vi "Remove INI Keys.vi"(8 "error in (no error)":errorcluster, 10 "Keys to remove":T1[](array[typedef]), 11 "INI file path":path) -> (0 "error out":errorcluster, 3 "Errors":string[](array[string]))   [LabVIEW 2016, in "RT Management.lvlib"]
doc: "Removes INI keys. If a key is the last one under a section and is removed, the section is left alone."
uses:
  RT Management.lvlib
  controls/INI key.ctl
  <vilib>/Utility/config.llb/NI_LVConfig.lvlib
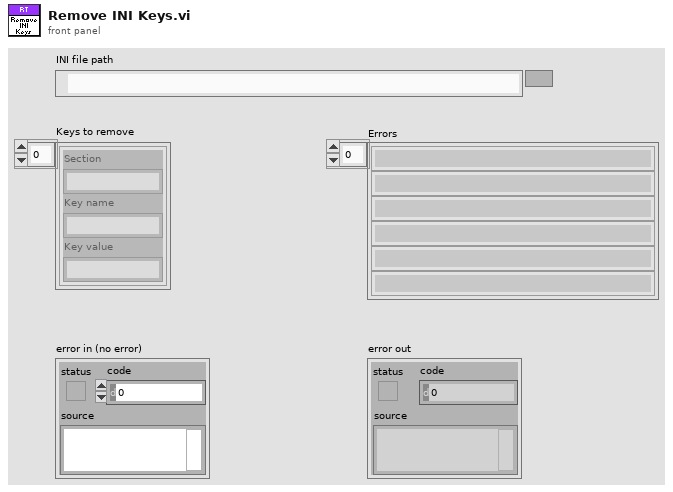
[diagram p1: front panel]
types:
  T1 = typedef "RT Management.lvlib/INI key.ctl" = cluster{"Section":string, "Key name":string, "Key value":string}
  T2 = typedef "NI_LVConfig.lvlib/Config Data RefNum.ctl" = refnum<k1>
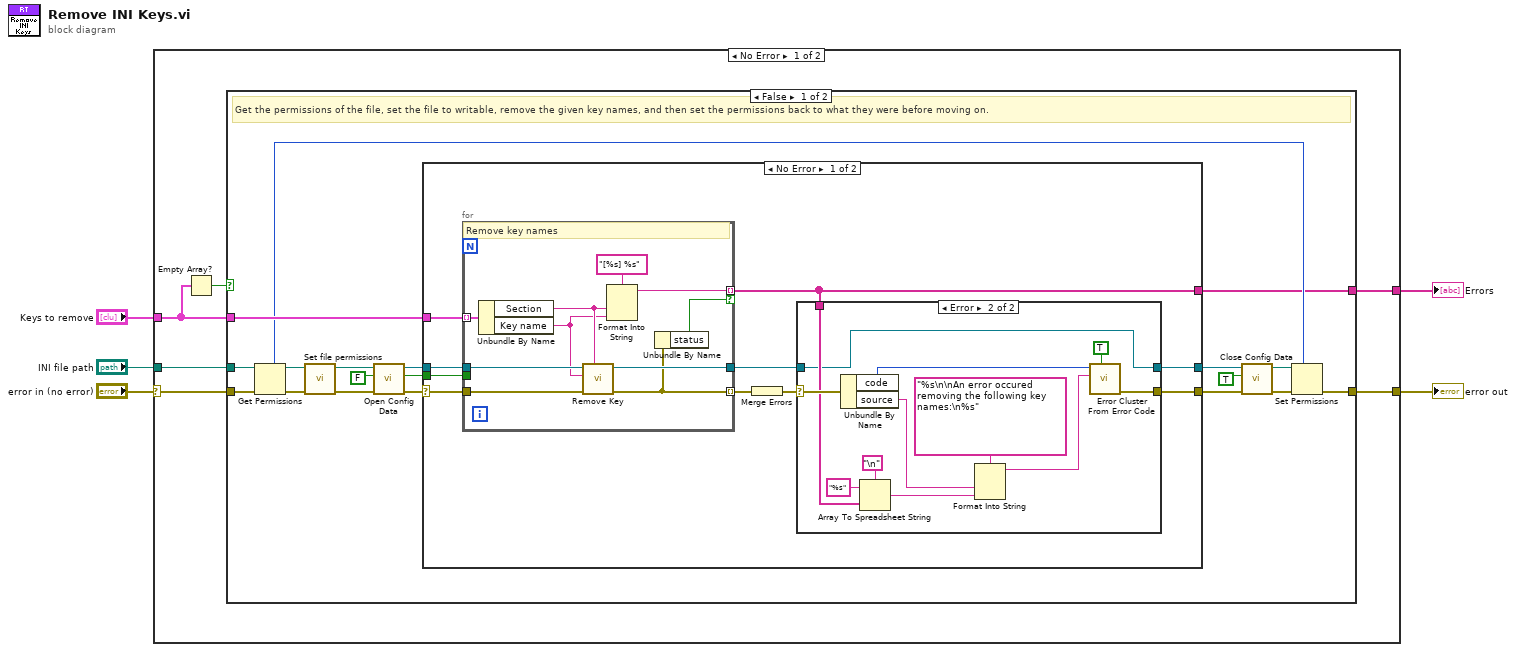
[diagram p0: block diagram]
diagram:
  n1 = case shown="No Error" "error in (no error)" {
    selector: "error in (no error)" -> [w7 w68]
    tunnel: "INI file path" -> [w11 _]
    tunnel: "Keys to remove" -> [w10 _]
    tunnel: [w8 w68] -> w3
    tunnel: [w6 _] -> w1
    frame No Error {
      n2 = Empty Array?(array=w10) -> (empty?=w9:bool)
      n3 = case shown="False" w9 {
        tunnel: w11 -> [w19 _]
        tunnel: w10 -> [w26 _]
        tunnel: [w16 w67] -> w8
        tunnel: w7 -> [w20 w67]
        tunnel: [w12 _] -> w6
        frame False {
          # "Get the permissions of the file, set the file to writable, remove the given key names, and then set the permissions back to what they were before moving on."
          n4 = Get Permissions(8:w20, 11:w19) -> (0:w13:errorcluster, 3:w14:path, 5:w15:i16)  [unwired: 2 out]
          n5 = call "Set file permissions.vi"("error in"=w13, "Path"=w14) -> ("error out"=w22:errorcluster, "Path Out"=w21:path)  [unwired: 8 in]
          n6 = call <vilib>:"Open Config Data.vi"("error in (no error)"=w22, "create file if necessary (T)"=FALSE, "configuration file path"=w21) -> ("error out"=w27:errorcluster, "file created?"=w29:bool, "refnum"=w28:T2)  [unwired: 6 in]
          n7 = case shown="No Error" w27 {
            selector: w27 -> [w37 w66]
            tunnel: w26 -> [w40 _]
            tunnel: w29 -> [w39 _]
            tunnel: w28 -> [w38 w65]
            tunnel: [w32 w66] -> w24
            tunnel: [w33 w65] -> w25
            tunnel: [w31 _] -> w12
            frame No Error {
              n8 = for {
                tunnel: w40 -> [w62] mode=indexing
                tunnel: w37 -> [w64]
                tunnel: w39 -> [_]
                tunnel: w38 -> [w63]
                tunnel: [w61] -> w34
                tunnel: [w56] -> w36 mode=indexing
                tunnel: [w57] -> w31 mode=indexing if=w55
                # "Remove key names"
                n9 = Unbundle By Name(w62) -> ("Section"=w59:string, "Key name"=w58:string)
                n10 = call <vilib>:"Remove Key.vi"("section"=w59, "error in (no error)"=w64, "key"=w58, "refnum"=w63) -> ("error out"=w56:errorcluster, "refnum out"=w61:T2)  [unwired: 5 in, 1 out]
                n11 = Format Into String(format string="[%s] %s", w59, w58) -> (resulting string=w57:string)  [unwired: 2 in, 1 out]
                n12 = Unbundle By Name(w56) -> ("status"=w55:bool)
              }
              n13 = Merge Errors(w36) -> (w35:errorcluster)
              n14 = case shown="Error" w35 {
                selector: w35 -> [w41 w53]
                tunnel: w34 -> [w42 w46]
                tunnel: [w42 w46] -> w33
                tunnel: [w41 w54] -> w32
                tunnel: w31 -> [_ w51]
                frame No Error {
                }
                frame Error {
                  n15 = Unbundle By Name(w53) -> ("code"=w52:i32, "source"=w43:string)
                  n16 = Array To Spreadsheet String(delimiter (Tab)="\n", array=w51, 3:"%s" ("format string")) -> (spreadsheet string=w44:string)
                  n17 = Format Into String(format string="%s\n\nAn error occured removing the following key names:\n%s", w43, w44) -> (resulting string=w47:string)  [unwired: 2 in, 1 out]
                  n18 = call <vilib>:"Error Cluster From Error Code.vi"("show call chain? (False)"=TRUE, "error message (\"\")"=w47, "error code (0)"=w52) -> ("error out"=w54:errorcluster)  [unwired: 6 in]
                }
              }
            }
            frame Error {
              # "Something went wrong with getting the file permissions, setting the file to writable, or the file doesn't exist."
            }
          }
          n19 = call <vilib>:"Close Config Data.vi"("error in (no error)"=w24, "write file if changed (T)"=TRUE, "refnum"=w25) -> ("error out"=w18:errorcluster, "file path"=w17:path)  [unwired: 7 in]
          n20 = Set Permissions(7:w15, 8:w18, 11:w17) -> (0:w16:errorcluster)  [unwired: 2 in, 1 out]
        }
        frame True {
          # "The Keys to remove array control is empty."
        }
      }
    }
    frame Error {
    }
  }
  "error out" <- w3
  "Errors" <- w1
